vi "PathPlanner_ConstraintsZone_GetAll.vi"(11 "ConstraintsZone":T2) -> (1 "Constraints":T1, 2 "maxWaypointPos":dbl, 3 "minWaypointPos":dbl)   [LabVIEW 2019, in "PathPlanner24.lvlib"]
doc: "Get the elements of the constraints zone cluster.\n \nInputs:\n -- ConstraintsZone - cluster - Data structure containing constraints zone.\n\nOutputs:\n -- minWayPointPos - double - Waypoint relative starting position\n -- maxWayPointPos - double - Waypoint relative end position\n -- Constaints -- cluster -- Constraints to apply within this region."
uses:
  PathPlanner24.lvlib
  TypeDef/PathPlannerConstraintsZone.ctl
  TypeDef/PathPlannerPathConstraints.ctl
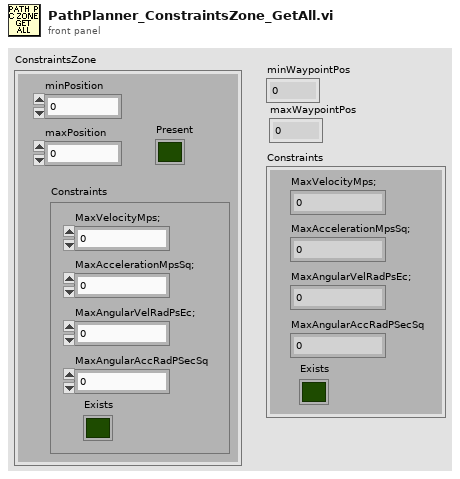
[diagram p1: front panel]
types:
  T1 = typedef "PathPlanner24.lvlib/PathPlannerPathConstraints.ctl" = cluster{"MaxVelocityMps;":dbl, "MaxAccelerationMpsSq;":dbl, "MaxAngularVelRadPsEc;":dbl, "MaxAngularAccRadPSecSq":dbl, "Exists":bool}
  T2 = typedef "PathPlanner24.lvlib/PathPlannerConstraintsZone.ctl" = cluster{"minPosition":dbl, "maxPosition":dbl, "Constraints":T1, "Present":bool}
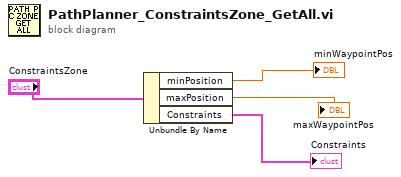
[diagram p0: block diagram]
diagram:
  n1 = Unbundle By Name("ConstraintsZone") -> ("minPosition"=→"minWaypointPos":dbl, "maxPosition"=→"maxWaypointPos":dbl, "Constraints"=→"Constraints":T1)
